vi "motion_server.vi"() -> ()   [LabVIEW 2024]
uses:
  motion_command.ctl
  motion_status.ctl
  <vilib>/Platform/TimedLoop/XDataNode/timing_clust.ctl
  <vilib>/Platform/TimedLoop/XDataNode/nitl_modes.ctl
  <vilib>/Platform/TimedLoop/XDataNode/wakeup.ctl
  <vilib>/Platform/TimedLoop/XDataNode/XDataNode.xnode
  <vilib>/Platform/TimedLoop/XDataNode/XDNodeRunTimeDep.lvlib
  <instrlib>/Trio Motion/Trio Motion Library.lvlib
panel:
  out "Homing fault":bool
  out "Home position":dbl[](array[numeric])
  out "End transform":dbl[](array[numeric])
  in  "Home":bool
  out "Motion status":T1={"Axis names"=["X", "Y", "Z", "Rx", "Ry", "Rz"], "Axis positions"=[], "Pose"=[], "Timestamp"=0, "Ready"=FALSE, "Stopped"=FALSE} {"Pose" format="%#.4f"; "Axis positions" format="%#.4f"}
  out "Stopped":bool
  in  "Emergency stop":bool
  in  "Home found":bool
  out "Command":T2={"Position"=[0.0, 0.0, 0.0, 0.0, 0.0, 0.0], "Axis enable"=[TRUE, TRUE, TRUE, TRUE, TRUE, TRUE], "Mode"=enum."Absolute axis", "Timestamp"=0}
  in  "Set origin":bool
  in  "stop":bool
  # "Motion server"
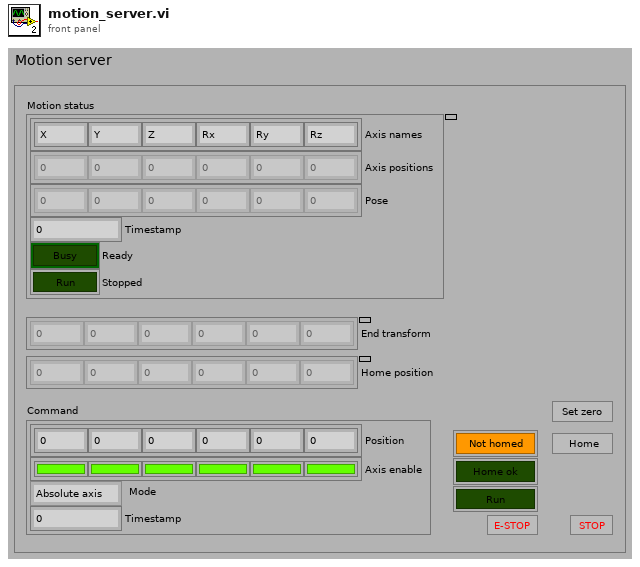
[diagram p1: front panel]
types:
  T1 = typedef "motion_status.ctl" = cluster{"Axis names":string[], "Axis positions":dbl[], "Pose":dbl[], "Timestamp":u32, "Ready":bool, "Stopped":bool}
  T2 = typedef "motion_command.ctl" = cluster{"Position":dbl[], "Axis enable":bool[], "Mode":enum16{"Absolute axis", "Relative axis", "Pose"}, "Timestamp":u32}
  T3 = typedef "XDNodeRunTimeDep.lvlib/timing_clust.ctl" = cluster{"Expected End [f-1]":u64, "Actual End [f-1]":u64, "Finished Late? [f-1]":bool, "Expected End [i-1]":u64, "Actual End [i-1]":u64, "Finished Late? [i-1]":bool, "Expected Start [i]":u64, "Actual Start [i]":u64, "Expected Start [f]":u64, "Actual Start [f]":u64, "Source Name":string, "Structure Name":string, "Period":i64, "Deadline":i64, "Offset":i64, "Start":i64, "Priority":i32, "Timeout":i32, "Mode":T4, "Wakeup Reason":T5, "Error":errorcluster, "Source Type":string, "Secondary Source Type":string, "Global End Time":u64, "Global Start Time":u64, "Frame Duration":u64, "Iteration Duration":u64, "Assigned CPU":i32, "I/O Scan Engine Mode":u32}
  T4 = typedef "XDNodeRunTimeDep.lvlib/nitl_modes.ctl" = enum32{"No Change", "Process missed periods, maintain original phase", "Discard missed periods, maintain original phase", "Process missed periods, ignore original phase", "Discard missed periods, ignore original phase"}
  T5 = typedef "XDNodeRunTimeDep.lvlib/wakeup.ctl" = enum32{"Normal", "Aborted", "Asynchronous wakeup", "Timing source error", "Timed loop error", "Timeout"}
  T6 = cluster{"HOMED":dbl, "BUSY":dbl, "ESTOP":dbl, "FAULT":dbl, "FAULT_AXIS":dbl, "STATE":dbl, "CUR_AXIS":dbl}
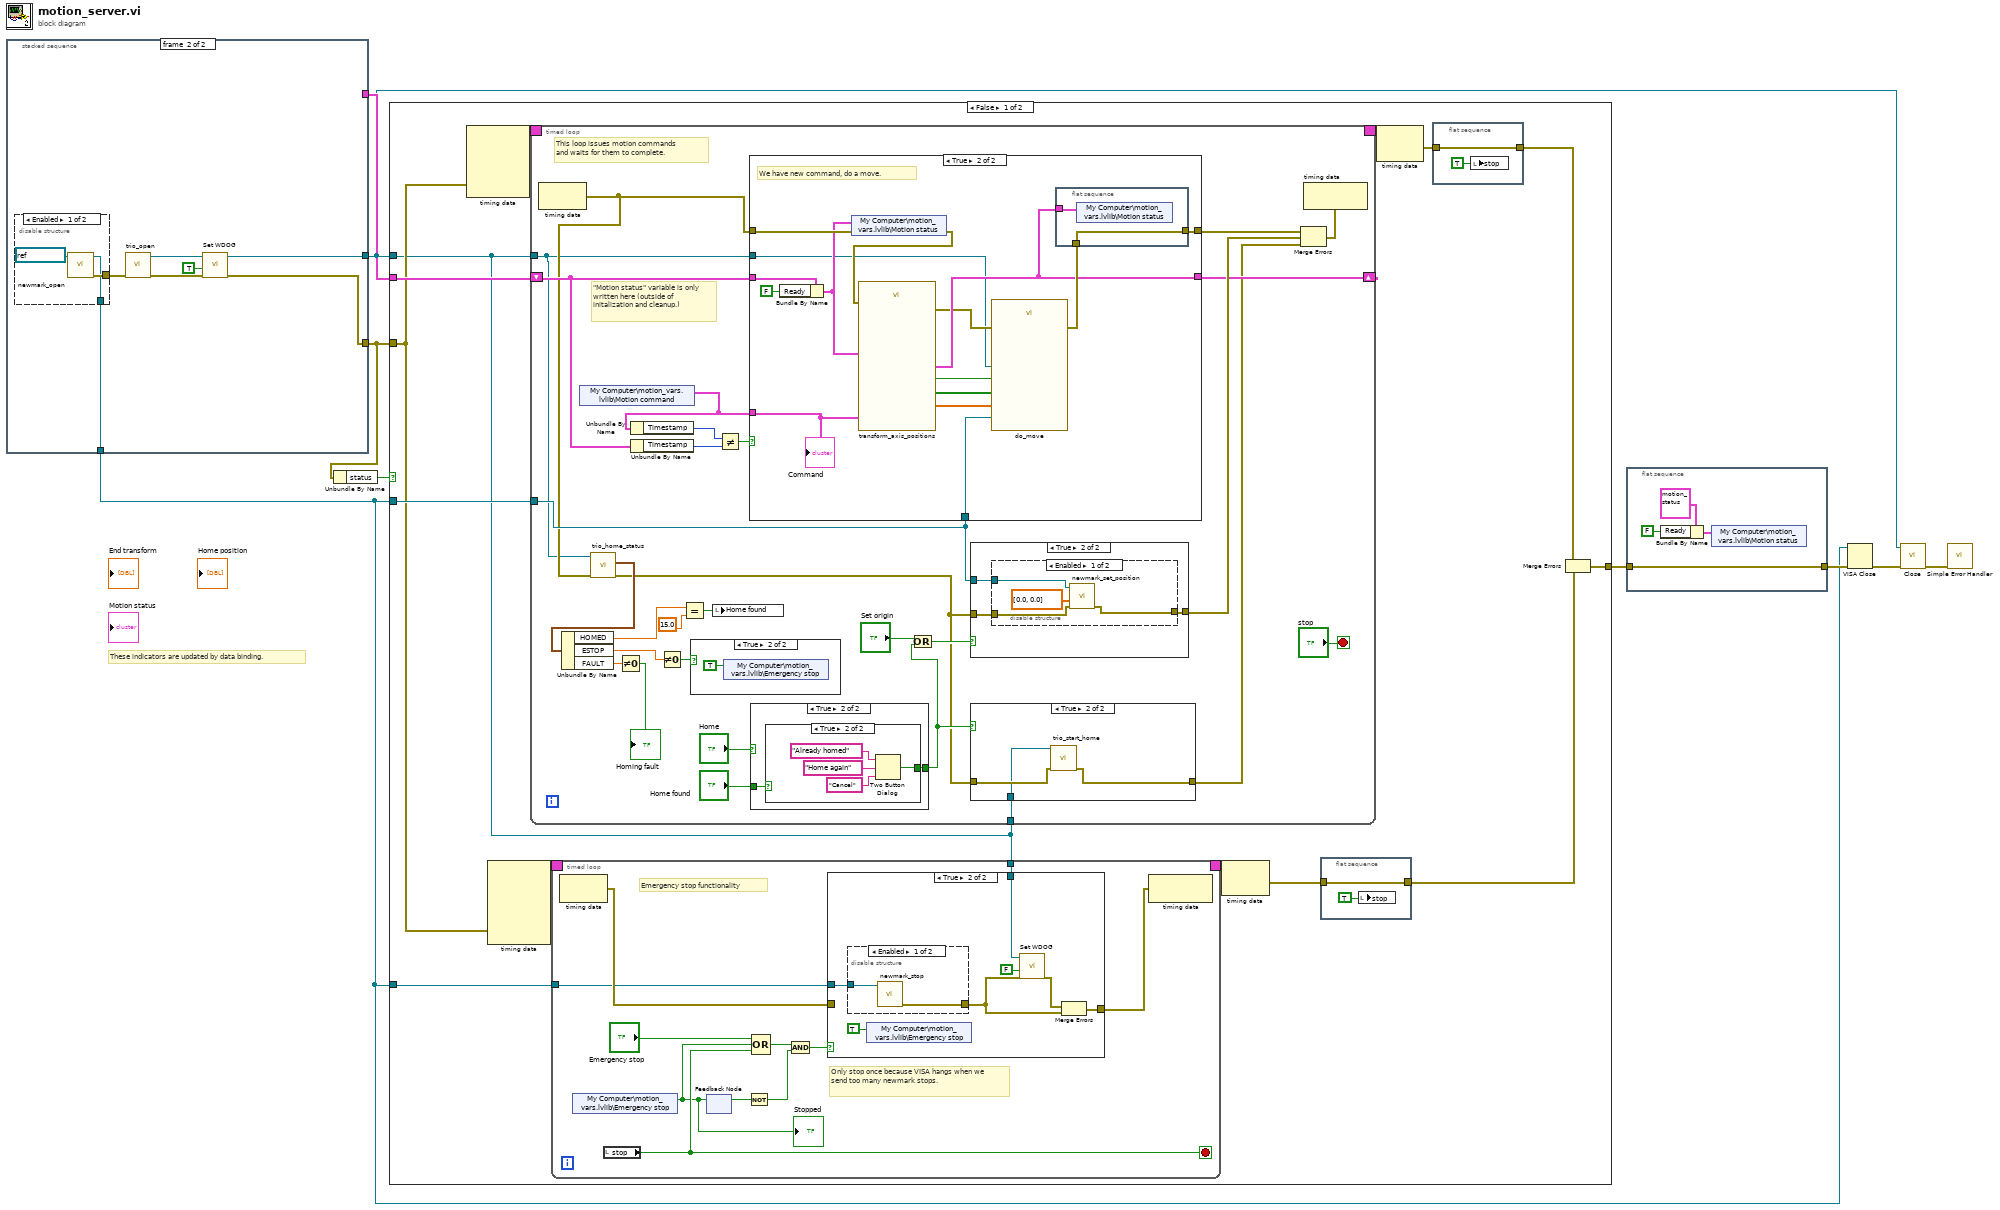
[diagram p0: block diagram]
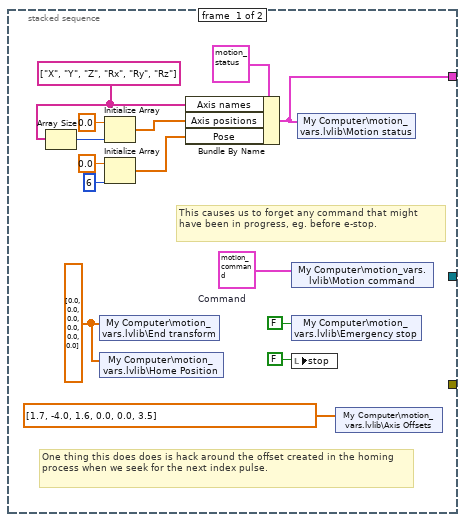
[diagram p2: hidden frame]
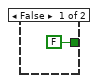
[diagram p6: hidden frame]
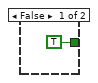
[diagram p7: hidden frame]
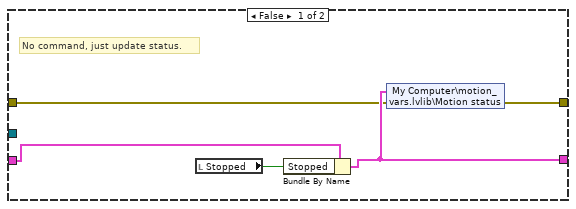
[diagram p12: hidden frame]
diagram:
  # "These indicators are updated by data binding."
  n1 = stacked-sequence {
    tunnel: [_ w26] -> w5
    tunnel: [w13 _] -> w6
    tunnel: [_ w29] -> w4
    tunnel: [_ w25] -> w1
    frame #0 {
      w10 = T2 {"Position"=[0.0, 0.0, 0.0, 0.0, 0.0, 0.0], "Axis enable"=[TRUE, TRUE, TRUE, TRUE, TRUE, TRUE], "Mode"=enum."Absolute axis", "Timestamp"=0}  # Command
      w14 = string[] ["X", "Y", "Z", "Rx", "Ry", "Rz"] ("Axis names")
      w12 = dbl[] [0.0, 0.0, 0.0, 0.0, 0.0, 0.0] ("End transform")
      # "This causes us to forget any command that might have been in progress, eg. before e-stop."
      # "One thing this does does is hack around the offset created in the homing process when we seek for the next index pulse."
      n2 = Array Size(array=w14) -> (size(s)=w22:i32)
      n3 = shared-variable "My Computer\\motion_vars.lvlib\\End transform"(w12) -> ()  [unwired: 1 in, 1 out]
      n4 = shared-variable "My Computer\\motion_vars.lvlib\\Home Position"(w12) -> ()  [unwired: 1 in, 1 out]
      n5 = Initialize Array(0.0, w22) -> (w20:dbl[])
      n6 = Initialize Array(0.0, 6 ("dimension size")) -> (w17:dbl[])
      n7 = Bundle By Name(cluster=T1 {"Axis names"=["X", "Y", "Z", "Rx", "Ry", "Rz"], "Axis positions"=[], "Pose"=[], "Timestamp"=0, "Ready"=TRUE, "Stopped"=FALSE} ("Motion status"), "Axis names"=w14, "Axis positions"=w20, "Pose"=w17) -> (w13:T1)
      n8 = shared-variable "My Computer\\motion_vars.lvlib\\Motion command"(w10) -> ()  [unwired: 1 in, 1 out]
      n9 = shared-variable "My Computer\\motion_vars.lvlib\\Emergency stop"(FALSE ("Emergency stop")) -> ()  [unwired: 1 in, 1 out]
      n10 = local write "stop"(FALSE ("stop")) -> ()
      n11 = shared-variable "My Computer\\motion_vars.lvlib\\Motion status"(w13) -> ()  [unwired: 1 in, 1 out]
      n12 = shared-variable "My Computer\\motion_vars.lvlib\\Axis Offsets"(dbl[] [1.7, -4.0, 1.6, 0.0, 0.0, 3.5] ("Axis offsets")) -> ()  [unwired: 1 in, 1 out]
    }
    frame #1 {
      n13 = disable-structure shown="Enabled" {
        disable-tunnel: [w33 _] -> w30
        disable-tunnel: [w32 _] -> w29
        frame Enabled {
          n14 = call "newmark_open.vi"("VISA Refnum in"=refnum<visa-resource-name> "COM3") -> ("error out"=w33:errorcluster, "VISA Refnum out"=w32:refnum<visa-resource-name>)  [unwired: 9 in]
        }
        frame Disabled {
        }
      }
      n15 = call "trio_open.vi"("error in"=w30) -> ("error out"=w27:errorcluster, "reference out"=w28:refnum<k7>)  [unwired: 9 in]
      n16 = call <instrlib>:"Set WDOG.vi"("error in (no error)"=w27, "WDOG (ON)"=TRUE, "reference in"=w28) -> ("error out"=w26:errorcluster, "reference out"=w25:refnum<k7>)  [unwired: 6 in, 1 out]
    }
  }
  n17 = Unbundle By Name(w5) -> ("status"=w9:bool)
  n18 = case shown="False" w9 {
    tunnel: w5 -> [w39 w166]
    tunnel: w4 -> [w43 _]
    tunnel: [w42 w166] -> w8
    tunnel: w6 -> [w41 _]
    tunnel: w4 -> [w40 _]
    tunnel: w1 -> [w34 _]
    frame False {
      n19 = node-c288(w39) -> (w47:T3)  [unwired: 3 in]
      n20 = node-c288(w39) -> (w45:T3)  [unwired: 4 in]
      n21 = timed-loop {
        tunnel: w43 -> [w107]
        timing: w47 -> [_]
        timing-out: [_] -> w46
        shift-right: [w105] -> _
        shift-left: w41 -> [w98]
        tunnel: w34 -> [w88]
        tunnel: w34 -> [w87]
        stop <- "stop" stop-if-true
        # "\"Motion status\" variable is only written here (outside of initalization and cleanup.)"
        # "This loop issues motion commands\nand waits for them to complete."
        n22 = node-c288() -> (w97:errorcluster)  [unwired: 1 in]
        n23 = shared-variable "My Computer\\motion_vars.lvlib\\Motion command"() -> (w102:T2)  [unwired: 1 in, 1 out]
        n24 = call "trio_home_status.vi"("error in"=w97, "reference in"=w88) -> ("Error out"=w83:errorcluster, "Status"=w96:T6)  [unwired: 7 in, 1 out]
        n25 = Unbundle By Name(w96) -> ("HOMED"=w95:dbl, "ESTOP"=w92:dbl, "FAULT"=w90:dbl)
        n26 = Not Equal To 0?(x=w90) -> (x != 0?=→"Homing fault":bool)
        n27 = Unbundle By Name(w102) -> ("Timestamp"=w103:u32)
        n28 = Unbundle By Name(w98) -> ("Timestamp"=w104:u32)
        n29 = Not Equal To 0?(x=w92) -> (x != 0?=w91:bool)
        n30 = Equal?(x=w95, y=15.0) -> (x = y?=w93:bool)
        n31 = case shown="True" w91 {
          frame False {
          }
          frame True {
            n32 = shared-variable "My Computer\\motion_vars.lvlib\\Emergency stop"(TRUE ("Emergency stop")) -> ()  [unwired: 1 in, 1 out]
          }
        }
        n33 = local write "Home found"(w93) -> ()
        n34 = Not Equal?(x=w103, y=w104) -> (x != y?=w106:bool)
        n35 = case shown="True" w106 {
          tunnel: w107 -> [_ w153]
          tunnel: [w134 w150] -> w110
          tunnel: w98 -> [w138 w152]
          tunnel: [w136 w148] -> w105
          tunnel: w97 -> [w135 w147]
          tunnel: w102 -> [_ w140]
          tunnel: w88 -> [_ w139]
          frame False {
            # "No command, just update status."
            n36 = local read "Stopped"() -> (w137:bool)
            n37 = Bundle By Name(cluster=w138, "Stopped"=w137) -> (w136:T1)
            n38 = shared-variable "My Computer\\motion_vars.lvlib\\Motion status"(w136, error in=w135) -> (error out=w134:errorcluster)
          }
          frame True {
            # "We have new command, do a move."
            n39 = Bundle By Name(cluster=w152, "Ready"=FALSE) -> (w141:T1)
            n40 = shared-variable "My Computer\\motion_vars.lvlib\\Motion status"(w141, error in=w147) -> (error out=w142:errorcluster)
            n41 = call "transform_axis_positions.vi"("Current status"=w141, "error in"=w142, "Command"=w140) -> ("error out"=w143:errorcluster, "Absolute"=w146:bool, "Axis positions"=w144:dbl[], "Axis enable"=w145:bool[], "Final status"=w148:T1)  [unwired: 4 in]
            n42 = call "do_move.vi"("Trio handle"=w139, "Absolute"=w146, "error in"=w143, "Axis positions"=w144, "Axis enable"=w145, "Newmark handle"=w153) -> ("error out"=w149:errorcluster)  [unwired: 5 in]
            n43 = flat-sequence {
              tunnel: [w154] -> w150
              tunnel: w149 -> [w154]
              tunnel: w148 -> [w155]
              frame #0 {
                n44 = shared-variable "My Computer\\motion_vars.lvlib\\Motion status"(w155) -> ()  [unwired: 1 in, 1 out]
              }
            }
            "Command" <- w140
          }
        }
        n45 = case shown="True" "Home" {
          tunnel: "Home found" -> [_ w114]
          tunnel: [FALSE ("T button?") w113] -> w84
          frame False {
          }
          frame True {
            n46 = case shown="True" w114 {
              tunnel: [TRUE ("T button?") w116] -> w113
              frame False {
              }
              frame True {
                n47 = Two Button Dialog(message="Already homed", 1:"Cancel" ("F button name (\"Cancel\")"), 2:"Home again" ("T button name (\"OK\")")) -> (T button?=w116:bool)
              }
            }
          }
        }
        n48 = Or(x="Set origin", y=w84) -> (x .or. y?=w99:bool)
        n49 = case shown="True" w99 {
          tunnel: w107 -> [_ w128]
          tunnel: w83 -> [w125 w127]
          tunnel: [w125 w126] -> w108
          frame False {
          }
          frame True {
            n50 = disable-structure shown="Enabled" {
              disable-tunnel: w128 -> [w132 _]
              disable-tunnel: w127 -> [w130 w133]
              disable-tunnel: [w129 w133] -> w126
              frame Enabled {
                n51 = call "newmark_set_position.vi"("error in"=w130, "Axis positions"=dbl[] [0.0, 0.0], "VISA Refnum in"=w132) -> ("error out"=w129:errorcluster)  [unwired: 7 in, 1 out]
              }
              frame Disabled {
              }
            }
          }
        }
        n52 = case shown="True" w84 {
          tunnel: w83 -> [w121 w124]
          tunnel: [w121 w123] -> w101
          tunnel: w87 -> [_ w122]
          frame False {
          }
          frame True {
            n53 = call "trio_start_home.vi"("error in"=w124, "reference in"=w122) -> ("Error out"=w123:errorcluster)  [unwired: 8 in, 1 out]
          }
        }
        n54 = Merge Errors(w110, w108, w101) -> (w109:errorcluster)
        n55 = node-c288(w109) -> ()  [unwired: 1 out]
      }
      n56 = timed-loop {
        timing: w45 -> [_]
        timing-out: [_] -> w44
        tunnel: w40 -> [w60]
        tunnel: w34 -> [w52]
        stop <- w58 stop-if-true
        # "Emergency stop functionality"
        # "Only stop once because VISA hangs when we send too many newmark stops."
        n57 = node-c288() -> (w62:errorcluster)  [unwired: 1 in]
        n58 = shared-variable "My Computer\\motion_vars.lvlib\\Emergency stop"() -> (w53:bool)  [unwired: 1 in, 1 out]
        "Stopped" <- w53
        n59 = local read "stop"() -> (w58:bool)
        n60 = feedback-in #1(w53) -> ()
        n61 = feedback #1() -> (w55:bool)  [unwired: 1 in]
        n62 = Not(x=w55) -> (.not. x?=w56:bool)
        n63 = Compound Arithmetic op=OR("Emergency stop", w53, w58) -> (w57:bool)
        n64 = And(x=w57, y=w56) -> (x .and. y?=w54:bool)
        n65 = case shown="True" w54 {
          tunnel: w62 -> [w63 _]
          tunnel: [w63 w68] -> w61
          tunnel: w60 -> [_ w70]
          tunnel: w52 -> [_ w65]
          frame False {
          }
          frame True {
            n66 = disable-structure shown="Enabled" {
              disable-tunnel: w70 -> [w72 _]
              disable-tunnel: [w71 _] -> w67
              frame Enabled {
                n67 = call "newmark_stop.vi"("VISA Refnum in"=w72) -> ("error out"=w71:errorcluster)  [unwired: 9 in, 1 out]
              }
              frame Disabled {
              }
            }
            n68 = shared-variable "My Computer\\motion_vars.lvlib\\Emergency stop"(TRUE ("Emergency stop")) -> ()  [unwired: 1 in, 1 out]
            n69 = call <instrlib>:"Set WDOG.vi"("error in (no error)"=w67, "WDOG (ON)"=FALSE, "reference in"=w65) -> ("error out"=w64:errorcluster)  [unwired: 6 in, 2 out]
            n70 = Merge Errors(w64, w67) -> (w68:errorcluster)
          }
        }
        n71 = node-c288(w61) -> ()  [unwired: 1 out]
      }
      n72 = node-c288(w44) -> (w38:errorcluster)
      n73 = flat-sequence {
        tunnel: w38 -> [w50]
        tunnel: [w50] -> w37
        frame #0 {
          n74 = local write "stop"(TRUE ("stop")) -> ()
        }
      }
      n75 = node-c288(w46) -> (w36:errorcluster)
      n76 = flat-sequence {
        tunnel: w36 -> [w48]
        tunnel: [w48] -> w35
        frame #0 {
          n77 = local write "stop"(TRUE ("stop")) -> ()
        }
      }
      n78 = Merge Errors(w35, w37) -> (w42:errorcluster)
    }
    frame True {
    }
  }
  n79 = flat-sequence {
    tunnel: w8 -> [w170]
    tunnel: [w170] -> w7
    frame #0 {
      n80 = Bundle By Name(cluster=T1 {"Axis names"=["X", "Y", "Z", "Rx", "Ry", "Rz"], "Axis positions"=[], "Pose"=[], "Timestamp"=0, "Ready"=FALSE, "Stopped"=FALSE} ("Motion status"), "Ready"=FALSE ("Moving?")) -> (w168:T1)
      n81 = shared-variable "My Computer\\motion_vars.lvlib\\Motion status"(w168) -> ()  [unwired: 1 in, 1 out]
    }
  }
  n82 = VISA Close(VISA resource name=w4, error in (no error)=w7) -> (error out=w3:errorcluster)
  n83 = call <instrlib>:"Close.vi"("error in (no error)"=w3, "reference in"=w1) -> ("error out"=w2:errorcluster)  [unwired: 9 in]
  n84 = call <vilib>:"Simple Error Handler.vi"("error in (no error)"=w2) -> ()  [unwired: 4 in, 5 out]
